vi "ModeLED.vi"(1 "Locate LED":bool, 2 "Choose Hue":bool) -> (0 "LED Mode":T1(ring))   [LabVIEW 2020]
doc: "Determines the appropriate LED mode based on the robot state, driver inputs, and live deploy configuration."
uses:
  <vilib>/Rock Robotics/WPI/DriverStation/WPI_DriverStationRobotMode2.ctl
  GlobalDriverStationData.vi
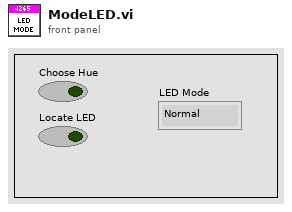
[diagram p1: front panel]
types:
  T1 = enum16{"Normal", "Party Mode", "Choose Hue", "Debug", "Locate LED", "Distance Rainbow"}
  T2 = typedef "WPI_DriverStationRobotMode2.ctl" = enum16{"Autonomous Disabled", "Autonomous Enabled", "Teleop Disabled", "Teleop Enabled", "Disconnected", "Finish", "Test Disabled", "Test Enabled", "Emergency Stopped"}
  T3 = enum16{"Center", "North", "NorthWest", "West", "SouthWest", "South", "SouthEast", "East", "NorthEast"}
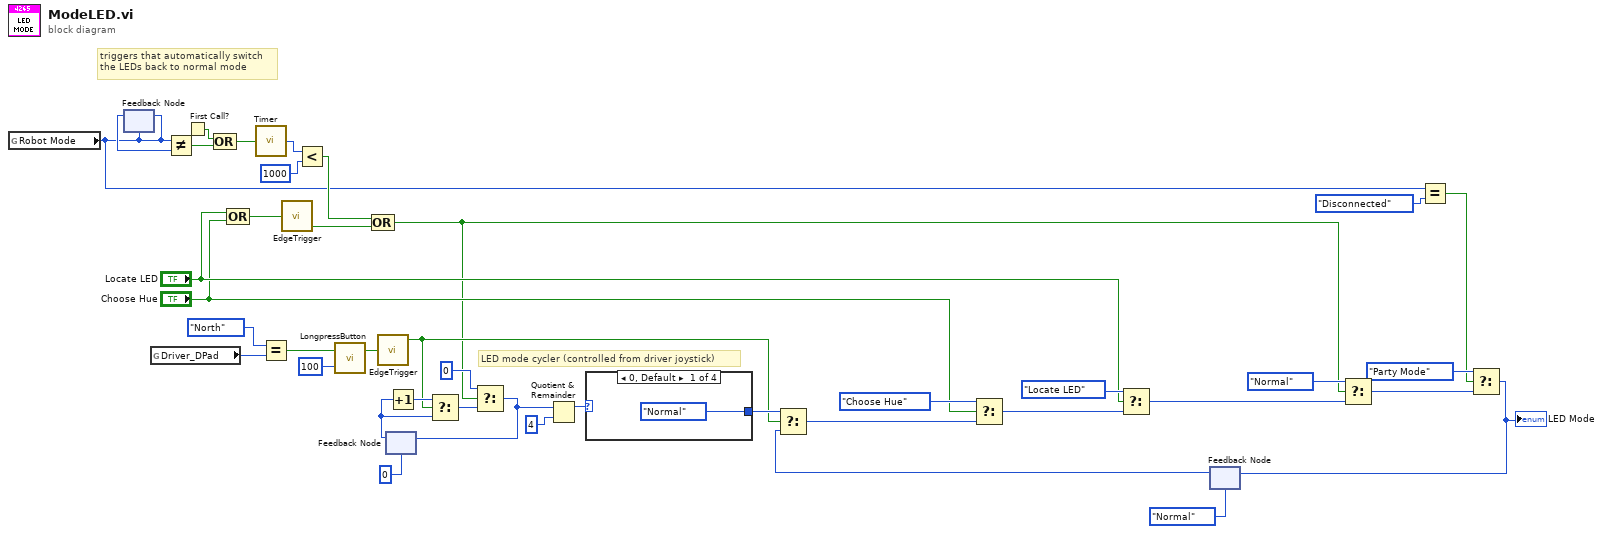
[diagram p0: block diagram]
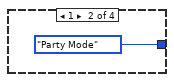
[diagram p2: hidden frame]
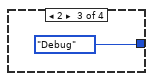
[diagram p3: hidden frame]
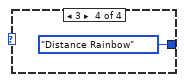
[diagram p4: hidden frame]
diagram:
  # "triggers that automatically switch\nthe LEDs back to normal mode"
  # "LED mode cycler (controlled from driver joystick)"
  n1 = global read "GlobalDriverStationData.vi" "Robot Mode"() -> (w3:T2)
  n2 = feedback #1(w3) -> (w41:T2)
  n3 = feedback-in #1(w3) -> ()
  n4 = global read "GlobalDriverStationData.vi" "Driver_DPad"() -> (w25:T3)
  n5 = Not Equal?(x=w3, y=w41) -> (x != y?=w29:bool)
  n6 = First Call?() -> (First Call?: T/F=w27:bool)
  n7 = Compound Arithmetic op=OR(w27, w29) -> (w28:bool)
  n8 = Compound Arithmetic op=OR("Locate LED", "Choose Hue") -> (w31:bool)
  n9 = call "Timer.vi"("Reset Timer"=w28) -> ("Time (ms)"=w37:u32)
  n10 = Equal?(x=T3."North", y=w25) -> (x = y?=w15:bool)
  n11 = call "EdgeTrigger.vi"("Input Signal"=w31) -> ("Falling Edge Trigger"=w30:bool)  [unwired: 2 out]
  n12 = Less?(x=w37, y=u32 1000) -> (x < y?=w35:bool)
  n13 = call "LongpressButton.vi"("Threshold (ms)"=u32 100, "Button"=w15) -> ("Longpress Button"=w13:bool)  [unwired: 1 out]
  n14 = Compound Arithmetic op=OR(w35, w30) -> (w7:bool)
  n15 = call "EdgeTrigger.vi"("Input Signal"=w13) -> ("Rising Edge Trigger"=w18:bool)  [unwired: 2 out]
  n16 = feedback #2(0) -> (w22:i32)
  n17 = Increment(x=w22) -> (x+1=w23:i32)
  n18 = Select(t=w23, s=w18, f=w22) -> (s? t:f=w12:i32)
  n19 = Select(t=0, s=w7, f=w12) -> (s? t:f=w11:i32)
  n20 = feedback-in #2(w11) -> ()
  n21 = Quotient & Remainder(x=w11, y=4) -> (x-y*floor(x/y)=w20:i32)  [unwired: 1 out]
  n22 = case shown="0, Default" w20 {
    tunnel: [T1."Normal" T1."Party Mode" T1."Debug" T1."Distance Rainbow"] -> w19
    frame 0, Default {
    }
    frame 1 {
    }
    frame 2 {
    }
    frame 3 {
    }
  }
  n23 = feedback #3(T1."Normal") -> (w16:T1)
  n24 = Select(t=w19, s=w18, f=w16) -> (s? t:f=w17:T1)
  n25 = Select(t=T1."Choose Hue", s="Choose Hue", f=w17) -> (s? t:f=w38:T1)
  n26 = Select(t=T1."Locate LED", s="Locate LED", f=w38) -> (s? t:f=w34:T1)
  n27 = Select(t=T1."Normal", s=w7, f=w34) -> (s? t:f=w5:T1)
  n28 = Equal?(x=w3, y=WPI_DriverStationRobotMode2."Disconnected") -> (x = y?=w2:bool)
  n29 = Select(t=T1."Party Mode", s=w2, f=w5) -> (s? t:f=w4:T1)
  "LED Mode" <- w4
  n30 = feedback-in #3(w4) -> ()
